vi "Unregister and Close Tasks.vi"(8 "error in":errorcluster) -> (0 "error out":errorcluster)   [LabVIEW 2021, in "NIDAQmxMeasurement.lvlib"]
doc: "This VI will get called as part of the TestStand ProcessCleanup sequence. It unregisters and destroys all DAQmx tasks in the Session Management Service."
uses:
  NIDAQmxMeasurement.lvlib
  <vilib>/Plug-In SDKs/Clients/Session Management V1/Session Reservation/Session Reservation.lvclass
  <vilib>/Plug-In SDKs/Sessions/niDAQmx/Session Management niDAQmx.lvlib
  <vilib>/Plug-In SDKs/Clients/Session Management V1/Session Reservation/Initialize and Close Session Behavior.ctl
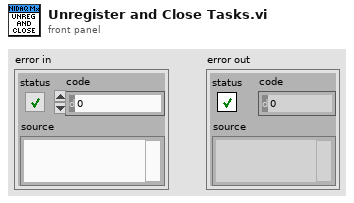
[diagram p1: front panel]
types:
  T1 = typedef "NI Session Management V1 Client.lvlib/Session Reservation.lvclass/Initialize and Close Session Behavior.ctl" = enum16{"Auto", "Initialize and Close", "Attach and Detach", "Initialize and Detach", "Attach and Close"}
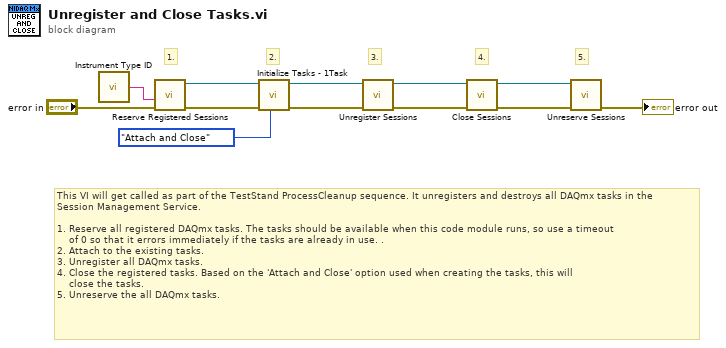
[diagram p0: block diagram]
diagram:
  # "3."
  # "5."
  # "4."
  # "2."
  # "1."
  # "This VI will get called as part of the TestStand ProcessCleanup sequence. It unregisters and destroys all DAQmx tasks in the\nSession Management Service.\n\n1. Reserve all registered DAQmx tasks. The tasks should be available when this code module runs, so use a timeout\n    of 0 so that it errors immediately if the tasks are already in use. .\n2. Attach to the existing tasks.\n3. Unregister all DAQmx tasks.\n4. Close the registered tasks. Based on the 'Attach and Close' option used when creating the tasks, this will\n    close the tasks.\n5. Unreserve the all DAQmx tasks."
  n1 = call <vilib>:"Instrument Type ID.vi"() -> ("instrument type id"=w2:string)  [unwired: 5 in]
  n2 = call <vilib>:"Reserve Registered Sessions.vi"("error in"="error in", "instrument type id"=w2) -> ("error out"=w11:errorcluster, "session reservation out"=w7:refnum<class "Session Reservation.lvclass">)  [unwired: 8 in]
  n3 = call <vilib>:"Initialize Tasks - 1Task.vi"("initialize and close session behavior"=Initialize_and_Close_Session_Behavior."Attach and Close", "error in"=w11, "session reservation in"=w7) -> ("error out"=w10:errorcluster, "session reservation out"=w6:refnum<class "Session Reservation.lvclass">)  [unwired: 5 in, 2 out]
  n4 = call <vilib>:"Unregister Sessions.vi"("error in"=w10, "session reservation in"=w6) -> ("error out"=w9:errorcluster, "session reservation out"=w5:refnum<class "Session Reservation.lvclass">)  [unwired: 8 in]
  n5 = call <vilib>:"Close Sessions.vi"("error in"=w9, "session reservation in"=w5) -> ("error out"=w8:errorcluster, "session reservation out"=w4:refnum<class "Session Reservation.lvclass">)  [unwired: 8 in]
  n6 = call <vilib>:"Unreserve Sessions.vi"("error in"=w8, "session reservation in"=w4) -> ("error out"=→"error out":errorcluster)  [unwired: 9 in]
